vi "Test Simple Connection.vi"() -> ()   [LabVIEW 2013]
uses:
  <vilib>/LabVIEW Open Source Project/MQTT Control Packets/Control Packets/CONNECT/CONNECT.lvclass
  <vilib>/LabVIEW Open Source Project/MQTT Control Packets/Control Packets/CONNACK/Connect Return Code -- enum.ctl
  MQTT_Connection/Connection/Connection.lvclass
  <vilib>/LabVIEW Open Source Project/MQTT Control Packets/Control Packets/PUBLISH/PUBLISH.lvclass
  <vilib>/LabVIEW Open Source Project/MQTT Control Packets/Control Packets/ControlPacket/ControlPacket.lvclass
  <vilib>/LabVIEW Open Source Project/MQTT Control Packets/Control Packets/CONNACK/CONNACK.lvclass
  <vilib>/LabVIEW Open Source Project/MQTT Control Packets/Control Packets/ControlPacket/ControlPacket.lvclass/ControlPacket.ctl
  <vilib>/LabVIEW Open Source Project/MQTT Control Packets/Control Packets/DISCONNECT/DISCONNECT.lvclass
  <vilib>/LabVIEW Open Source Project/MQTT Control Packets/Control Packets/MQTT_311/MQTTVersion.lvclass
  MQTT_TCP/Connection/TCPConnection.lvclass
  MQTT_LocalQueue/Connection/LocalQueueConnection.lvclass
panel:
  in  "Channel Under Test":T1(ring)
  in  "Range (max)":dbl=1.0
  out "randomNumber":dbl
  out "Topic":string
  out "connected":bool
  in  "Connect to Server":bool
  out "client":errorcluster
  out "server":errorcluster
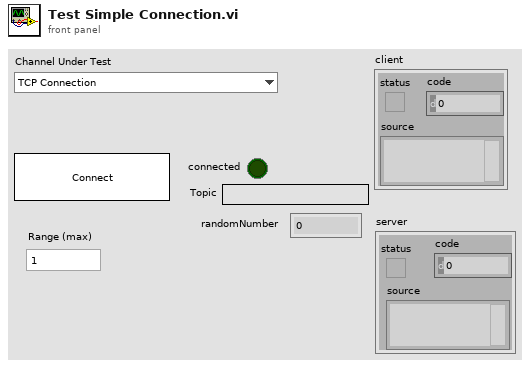
[diagram p1: front panel]
types:
  T1 = enum16{"TCP Connection", "Local Queue Connection"}
  T2 = cluster{"Packet":refnum<class "ControlPacket.lvclass">, "Direction":enum16{"In", "Out"}}
  T3 = cluster{"connected":refnum<user-event>, "Incoming Message":refnum<user-event>}
  T4 = cluster{"Connection":refnum<class "Connection.lvclass">, "Public Events":cluster{"connected":refnum<user-event>, "Incoming Message":refnum<user-event>}, "Payload":refnum<queue>}
  T5 = typedef "MQTT_Control_Packets.lvlib/CONNACK.lvclass/Connect Return Code -- enum.ctl" = enum16{"Connection accepted", "Unacceptable protocol version", "Identifier Rejected", "Server Unavailable", "Bad Username or Password", "Not Authorized"}
  T6 = enum16{"Standard", "Buffered", "CRLF", "Immediate"}
  T7 = typedef "MQTT_Control_Packets.lvlib/ControlPacket.lvclass/Control Packet Type -- enum.ctl" = enum16{"Reserved", "CONNECT", "CONNACK", "PUBLISH", "PUBACK", "PUBREC", "PUBREL", "PUBCOMP", "SUBSCRIBE", "SUBACK", "UNSUBSCRIBE", "UNSUBACK", "PINGREQ", "PINGRESP", "DISCONNECT", "AUTH"}
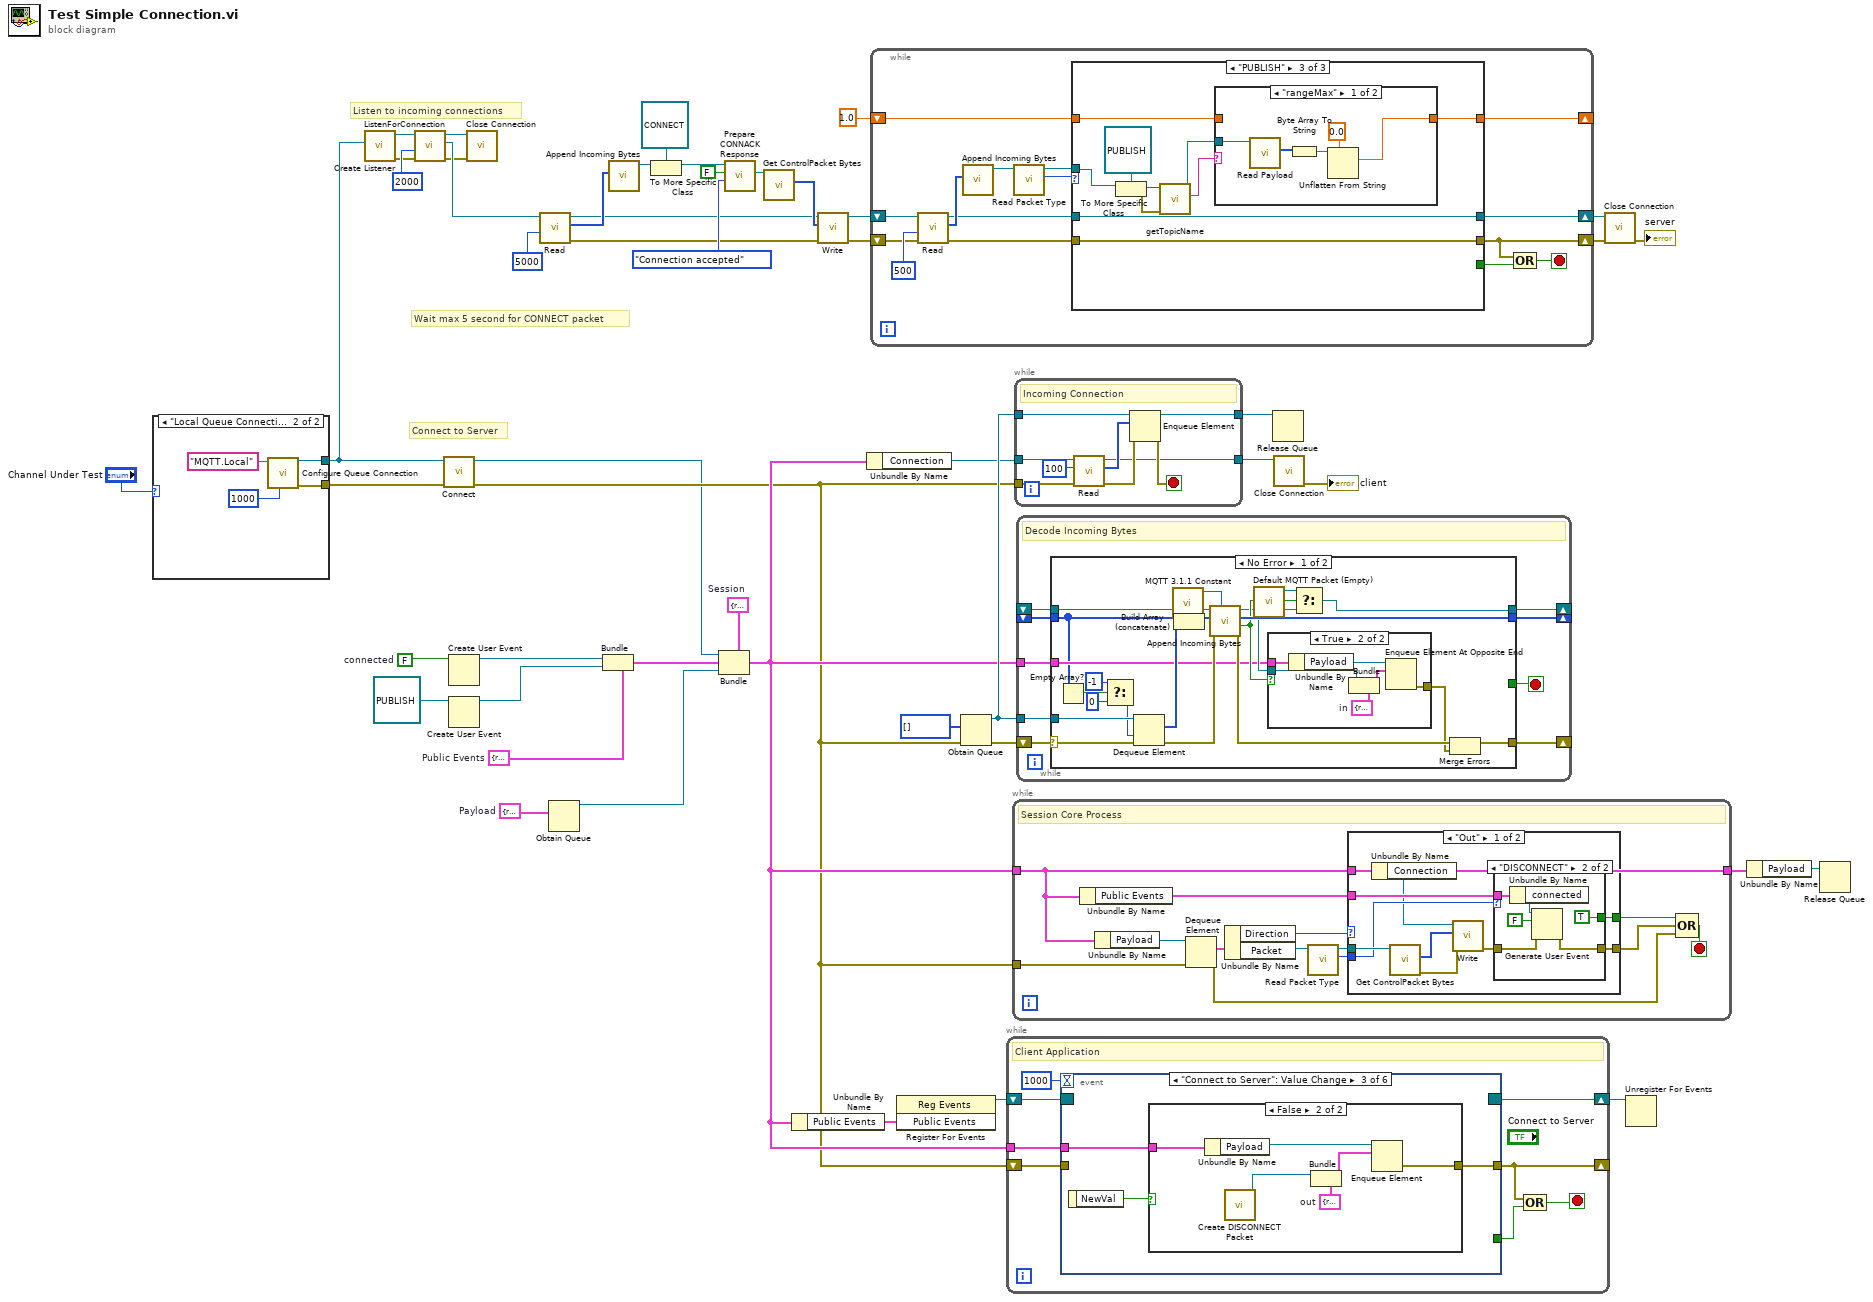
[diagram p0: block diagram]
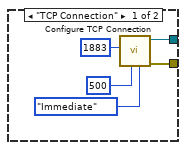
[diagram p2: hidden frame]
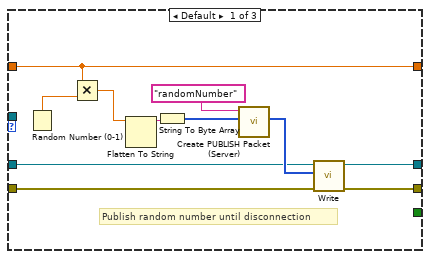
[diagram p3: hidden frame]
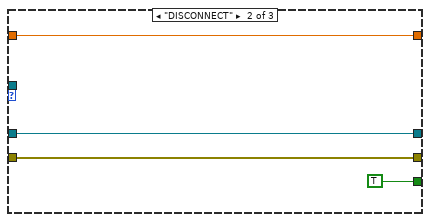
[diagram p4: hidden frame]
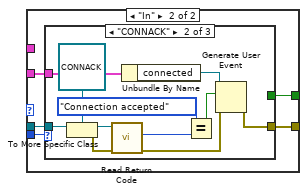
[diagram p7: hidden frame]
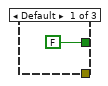
[diagram p8: hidden frame]
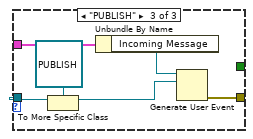
[diagram p9: hidden frame]
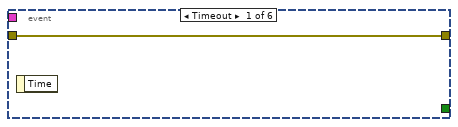
[diagram p10: hidden frame]
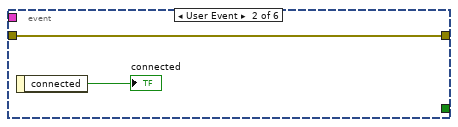
[diagram p11: hidden frame]
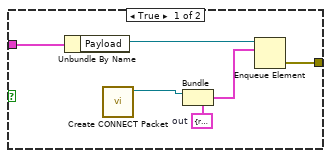
[diagram p12: hidden frame]
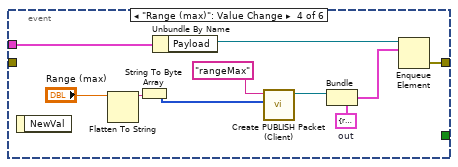
[diagram p13: hidden frame]
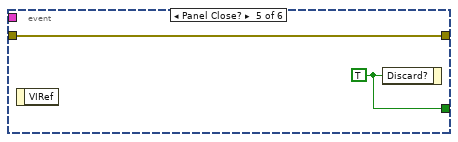
[diagram p14: hidden frame]
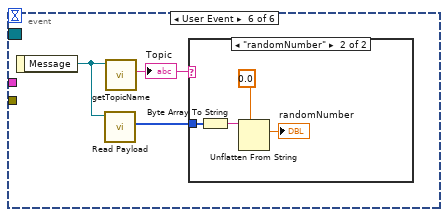
[diagram p15: hidden frame]
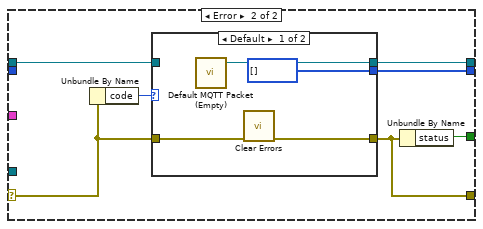
[diagram p18: hidden frame]
diagram:
  w21 = T2 {"Packet"=refnum, "Direction"=enum."In"}  # Payload
  w34 = T3 {"connected"=refnum, "Incoming Message"=refnum}  # Public Events
  w35 = FALSE  # connected
  w37 = T4 {"Connection"=refnum, "Public Events"={"connected"=refnum, "Incoming Message"=refnum}, "Payload"=refnum}  # Session
  # "Connect to Server"
  # "Listen to incoming connections"
  # "Wait max 5 second for CONNECT packet"
  n1 = case shown="\"Local Queue Connection\"" "Channel Under Test" {
    tunnel: [w52 w57] -> w9
    tunnel: [w51 w58] -> w2
    frame "TCP Connection" {
      n2 = call "Configure TCP Connection.vi"("Read Mode (Immediate)"=T6."Immediate" ("mode (standard)"), "timeout (5000ms)"=500 ("timeout (100ms)"), "remote port (80)"=u16 1883) -> ("error out"=w52:errorcluster, "TCPConnection"=w51:refnum<class "TCPConnection.lvclass">)  [unwired: 7 in]
    }
    frame "Local Queue Connection" {
      n3 = call "Configure Queue Connection.vi"("timeout (500 ms)"=1000 ("timeout (100ms)"), "Queue Name"="MQTT.Local") -> ("error out"=w57:errorcluster, "LocalQueueConnection"=w58:refnum<class "LocalQueueConnection.lvclass">)  [unwired: 8 in]
    }
  }
  n4 = call "Create Listener.vi"("Connection Configuration"=w2) -> ("error out"=w4:errorcluster, "Listener"=w8:refnum<class "Connection.lvclass">)  [unwired: 9 in]
  n5 = call "ListenForConnection.vi"("error in (no error)"=w4, "timeout (ms)"=2000 ("bytes to read (100)"), "Listener"=w8) -> ("error out"=w3:errorcluster, "Connection"=w5:refnum<class "Connection.lvclass">, "Listener out"=w6:refnum<class "Connection.lvclass">)  [unwired: 5 in, 1 out]
  n6 = call "Connect.vi"("error in (no error)"=w9, "Connection in"=w2) -> ("error out"=w11:errorcluster, "Connection out"=w10:refnum<class "Connection.lvclass">)  [unwired: 8 in]
  n7 = Create User Event(user event datatype=w35) -> (user event=w36:refnum<user-event>)  [unwired: 1 in, 1 out]
  n8 = Create User Event(user event datatype=refnum<class "PUBLISH.lvclass"> refnum ("Message")) -> (user event=w26:refnum<user-event>)  [unwired: 1 in, 1 out]
  n9 = call "Close Connection.vi"("error in (no error)"=w3, "Connection in"=w6) -> ()  [unwired: 8 in, 2 out]
  n10 = call "Read.vi"("timeout (1000 ms)"=5000 ("bytes to read (100)"), "TCPConnection in"=w5) -> ("error out"=w14:errorcluster, "Bytes"=w13:u8[], "TCPConnection out"=w12:refnum<class "Connection.lvclass">)  [unwired: 5 in, 2 out]
  n11 = Obtain Queue(element data type=w21) -> (queue out=w19:refnum<queue>)  [unwired: 4 in, 2 out]
  n12 = Bundle(cluster=w34, "connected"=w36, "Incoming Message"=w26) -> (w20:T3)
  n13 = call <vilib>:"Append Incoming Bytes.vi"("Incoming Packets"=w13) -> ("ControlPacket"=w50:refnum<class "ControlPacket.lvclass">)  [unwired: 7 in, 3 out]
  n14 = To More Specific Class(target class=refnum<class "CONNECT.lvclass"> refnum ("CONNECT in"), reference=w50) -> (specific class reference=w49:refnum<class "CONNECT.lvclass">)  [unwired: 1 in, 1 out]
  n15 = Bundle(cluster=w37, "Connection"=w10, "Public Events"=w20, "Payload"=w19) -> (w17:T4)
  n16 = call-dynamic "Prepare CONNACK Response.vi"("Return Code"=Connect_Return_Code_--_enum."Connection accepted", "Session Present"=FALSE, "CONNECT in"=w49) -> ("CONNACK response"=w46:refnum<class "CONNACK.lvclass">)  [unwired: 5 in, 3 out]
  n17 = call <vilib>:"Get ControlPacket Bytes.vi"("ControlPacket"=w46) -> ("Bytes Stream"=w47:u8[])  [unwired: 7 in, 3 out]
  n18 = Unbundle By Name(w17) -> ("Public Events"=w33:T3)
  n19 = call "Write.vi"("error in (no error)"=w14, "Bytes"=w47, "Connection in"=w12) -> ("error out"=w24:errorcluster, "Connection"=w25:refnum<class "Connection.lvclass">)  [unwired: 7 in]
  n20 = Unbundle By Name(w17) -> ("Connection"=w16:refnum<class "Connection.lvclass">)
  n21 = while {
    shift-right: [w66] -> w23
    shift-left: w25 -> [w71]
    shift-right: [w63] -> w22
    shift-left: w24 -> [w70]
    shift-right: [w61] -> _
    shift-left: 1.0 -> [w62]
    stop <- w64 stop-if-true
    n22 = call "Read.vi"("error in (no error)"=w70, "timeout (1000 ms)"=500 ("bytes to read (100)"), "TCPConnection in"=w71) -> ("error out"=w67:errorcluster, "Bytes"=w74:u8[], "TCPConnection out"=w68:refnum<class "Connection.lvclass">)  [unwired: 4 in, 2 out]
    n23 = call <vilib>:"Append Incoming Bytes.vi"("Incoming Packets"=w74) -> ("ControlPacket"=w73:refnum<class "ControlPacket.lvclass">)  [unwired: 7 in, 3 out]
    n24 = call <vilib>:"Read Packet Type.vi"("ControlPacket in"=w73) -> ("Control Packet Type"=w69:T7, "ControlPacket out"=w60:refnum<class "ControlPacket.lvclass">)  [unwired: 9 in]
    n25 = case shown="\"PUBLISH\"" w69 {
      tunnel: w68 -> [w81 w89 w99]
      tunnel: w67 -> [w78 w88 w98]
      tunnel: [w80 w89 w99] -> w66
      tunnel: [w79 w88 w98] -> w63
      tunnel: [_ TRUE _] -> w65
      tunnel: w62 -> [w75 w86 w92]
      tunnel: [w75 w86 w91] -> w61
      tunnel: w60 -> [_ _ w96]
      frame Default {
        # "Publish random number until disconnection"
        n26 = Random Number (0-1)() -> (number: 0 to 1=w77:dbl)
        n27 = Multiply(x=w75, y=w77) -> (x*y=w76:dbl)
        n28 = Flatten To String(anything=w76) -> (data string=w83:string)  [unwired: 3 in, 2 out]
        n29 = String To Byte Array(string=w83) -> (unsigned byte array=w84:u8[])
        n30 = call <vilib>:"Create PUBLISH Packet (Server).vi"("Payload"=w84, "Topic Name"="randomNumber") -> ("Bytes Stream"=w85:u8[])  [unwired: 6 in, 3 out]
        n31 = call "Write.vi"("error in (no error)"=w78, "Bytes"=w85, "Connection in"=w81) -> ("error out"=w79:errorcluster, "Connection"=w80:refnum<class "Connection.lvclass">)  [unwired: 7 in]
      }
      frame "DISCONNECT" {
      }
      frame "PUBLISH" {
        n32 = To More Specific Class(target class=refnum<class "PUBLISH.lvclass"> refnum ("event data"), reference=w96) -> (specific class reference=w94:refnum<class "PUBLISH.lvclass">, error out=w95:errorcluster)  [unwired: 1 in]
        n33 = call <vilib>:"getTopicName.vi"("error in (no error)"=w95, "PUBLISH in"=w94) -> ("Topic"=w93:string, "PUBLISH out"=w90:refnum<class "PUBLISH.lvclass">)  [unwired: 7 in, 1 out]
        n34 = case shown="\"rangeMax\"" w93 {
          tunnel: w92 -> [_ w105]
          tunnel: [w100 w105] -> w91
          tunnel: w90 -> [w104 _]
          frame "rangeMax" {
            n35 = call <vilib>:"Read Payload.vi"("ControlPacket in"=w104) -> ("Payload"=w101:u8[])  [unwired: 9 in, 1 out]
            n36 = Byte Array To String(unsigned byte array=w101) -> (string=w102:string)
            n37 = Unflatten From String(type=0.0, binary string=w102) -> (value=w100:dbl)  [unwired: 3 in, 2 out]
          }
          frame Default {
          }
        }
      }
    }
    n38 = Compound Arithmetic op=OR(w63, w65) -> (w64:bool)
  }
  n39 = register-events(w33) -> (reference out=w39:refnum<event-registration>)  [unwired: 2 in, 1 out]
  n40 = Obtain Queue(element data type=u8[] [] ("Remaining Packets"), error in (no error)=w11) -> (queue out=w43:refnum<queue>, error out=w41:errorcluster)  [unwired: 3 in, 1 out]
  n41 = while {
    shift-right: [w111] -> w38
    shift-left: w39 -> [w112]
    shift-right: [w109] -> _
    shift-left: w11 -> [w110]
    tunnel: w17 -> [w107]
    stop <- w108 stop-if-true
    # "Client Application"
    n42 = event shown="[2] \"Connect to Server\": Value Change" {
      selector: w112 -> [_ _ _ _ _ _]
      dyn-events: [_ _ _ _ _ _] -> w111
      timeout: 1000 -> [_ _ _ _ _ _]
      tunnel: [_ _ _ _ w143 _] -> w106
      tunnel: [w114 w116 w117 w140 w142 _] -> w109
      tunnel: w110 -> [w114 w116 _ _ w142 _]
      tunnel: w107 -> [_ _ w118 w141 _ _]
      event Timeout {
        n43 = event-data() -> ()  [unwired: 1 in, 1 out]
      }
      event User Event {
        n44 = event-data() -> ("connected"=→"connected":bool)  [unwired: 1 in]
      }
      event "Connect to Server": Value Change {
        n45 = event-data() -> ("NewVal"=w119:bool)  [unwired: 1 in]
        n46 = case shown="False" w119 {
          tunnel: w118 -> [w125 w131]
          tunnel: [w123 w129] -> w117
          frame True {
            w122 = T2 {"Packet"=refnum, "Direction"=enum."Out"}  # out
            n47 = Unbundle By Name(w125) -> ("Payload"=w124:refnum<queue>)
            n48 = call <vilib>:"Create CONNECT Packet.vi"() -> ("CONNECT"=w121:refnum<class "CONNECT.lvclass">)  [unwired: 9 in, 2 out]
            n49 = Bundle(cluster=w122, "Packet"=w121) -> (w120:T2)  [unwired: 1 in]
            n50 = Enqueue Element(queue=w124, element=w120) -> (error out=w123:errorcluster)  [unwired: 2 in, 2 out]
          }
          frame False {
            w126 = T2 {"Packet"=refnum, "Direction"=enum."Out"}  # out
            n51 = Unbundle By Name(w131) -> ("Payload"=w130:refnum<queue>)
            n52 = call <vilib>:"Create DISCONNECT Packet.vi"() -> ("DISCONNECT"=w128:refnum<class "DISCONNECT.lvclass">)  [unwired: 9 in, 2 out]
            n53 = Bundle(cluster=w126, "Packet"=w128) -> (w127:T2)  [unwired: 1 in]
            n54 = Enqueue Element(queue=w130, element=w127) -> (error out=w129:errorcluster)  [unwired: 2 in, 2 out]
          }
        }
      }
      event "Range (max)": Value Change {
        w138 = T2 {"Packet"=refnum, "Direction"=enum."Out"}  # out
        n55 = event-data() -> ()  [unwired: 1 in, 1 out]
        n56 = Flatten To String(anything="Range (max)") -> (data string=w134:string)  [unwired: 3 in, 2 out]
        n57 = String To Byte Array(string=w134) -> (unsigned byte array=w133:u8[])
        n58 = Unbundle By Name(w141) -> ("Payload"=w139:refnum<queue>)
        n59 = call <vilib>:"Create PUBLISH Packet (Client).vi"("Payload"=w133, "Topic Name"="rangeMax") -> ("PUBLISH"=w136:refnum<class "PUBLISH.lvclass">)  [unwired: 6 in, 3 out]
        n60 = Bundle(cluster=w138, "Packet"=w136) -> (w137:T2)  [unwired: 1 in]
        n61 = Enqueue Element(queue=w139, element=w137) -> (error out=w140:errorcluster)  [unwired: 2 in, 2 out]
      }
      event Panel Close? {
        w143 = TRUE ("Discard?")
        n62 = event-data() -> ()  [unwired: 1 in, 1 out]
        n63 = event-data("Discard?"=w143) -> ()  [unwired: 1 in, 1 out]
      }
      event User Event {
        n64 = event-data() -> ("Message"=w146:refnum<class "PUBLISH.lvclass">)  [unwired: 1 in]
        n65 = call <vilib>:"Read Payload.vi"("ControlPacket in"=w146) -> ("Payload"=w144:u8[])  [unwired: 9 in, 1 out]
        n66 = call <vilib>:"getTopicName.vi"("PUBLISH in"=w146) -> ("Topic"=w145:string)  [unwired: 8 in, 2 out]
        "Topic" <- w145
        n67 = case shown="\"randomNumber\"" w145 {
          tunnel: w144 -> [_ w149]
          frame "False", Default {
          }
          frame "randomNumber" {
            n68 = Byte Array To String(unsigned byte array=w149) -> (string=w148:string)
            n69 = Unflatten From String(type=0.0, binary string=w148) -> (value=→"randomNumber":dbl)  [unwired: 3 in, 2 out]
          }
        }
      }
    }
    n70 = Compound Arithmetic op=OR(w109, w106) -> (w108:bool)
  }
  n71 = while {
    tunnel: w17 -> [w152]
    tunnel: [w152] -> w32
    tunnel: w11 -> [w161]
    stop <- w157 stop-if-true
    # "Session Core Process"
    n72 = Unbundle By Name(w152) -> ("Public Events"=w151:T3)
    n73 = Unbundle By Name(w152) -> ("Payload"=w156:refnum<queue>)
    n74 = Dequeue Element(queue=w156, error in (no error)=w161) -> (element=w155:T2, error out=w158:errorcluster)  [unwired: 1 in, 2 out]
    n75 = Unbundle By Name(w155) -> ("Direction"=w153:enum16{"In", "Out"}, "Packet"=w154:refnum<class "ControlPacket.lvclass">)
    n76 = call <vilib>:"Read Packet Type.vi"("ControlPacket in"=w154) -> ("Control Packet Type"=w163:T7, "ControlPacket out"=w162:refnum<class "ControlPacket.lvclass">)  [unwired: 9 in]
    n77 = case shown="\"Out\"" w153 {
      tunnel: w163 -> [w169 w185]
      tunnel: w162 -> [w171 w184]
      tunnel: [w173 w183] -> w160
      tunnel: [w172 w182] -> w159
      tunnel: w152 -> [w170 _]
      tunnel: w151 -> [w168 w181]
      frame "Out" {
        n78 = Unbundle By Name(w170) -> ("Connection"=w167:refnum<class "Connection.lvclass">)
        n79 = call <vilib>:"Get ControlPacket Bytes.vi"("ControlPacket"=w171) -> ("error out"=w165:errorcluster, "Bytes Stream"=w166:u8[])  [unwired: 7 in, 2 out]
        n80 = call "Write.vi"("error in (no error)"=w165, "Bytes"=w166, "Connection in"=w167) -> ("error out"=w164:errorcluster)  [unwired: 7 in, 1 out]
        n81 = case shown="\"DISCONNECT\"" w169 {
          tunnel: [_ TRUE] -> w173
          tunnel: [w174 w178] -> w172
          tunnel: w164 -> [w174 w177]
          tunnel: w168 -> [_ w176]
          frame Default {
          }
          frame "DISCONNECT" {
            n82 = Unbundle By Name(w176) -> ("connected"=w175:refnum<user-event>)
            n83 = Generate User Event(user event=w175, event data cluster=FALSE ("event data"), error in=w177) -> (error out=w178:errorcluster)  [unwired: 1 in, 1 out]
          }
        }
      }
      frame "In" {
        n84 = case shown="\"CONNACK\"" w185 {
          tunnel: w184 -> [_ w197 w202]
          tunnel: [_ w192 w203] -> w182
          tunnel: [FALSE _ _] -> w183
          tunnel: w181 -> [_ w187 w199]
          frame Default {
          }
          frame "CONNACK" {
            n85 = To More Specific Class(target class=refnum<class "CONNACK.lvclass"> refnum ("CONNACK in"), reference=w197) -> (specific class reference=w195:refnum<class "CONNACK.lvclass">, error out=w190:errorcluster)  [unwired: 1 in]
            n86 = call <vilib>:"Read Return Code.vi"("error in (no error)"=w190, "CONNACK in"=w195) -> ("error out"=w191:errorcluster, "Return Code"=w194:T5)  [unwired: 7 in, 1 out]
            n87 = Unbundle By Name(w187) -> ("connected"=w188:refnum<user-event>)
            n88 = Equal?(x=Connect_Return_Code_--_enum."Connection accepted", y=w194) -> (x = y?=w193:bool)
            n89 = Generate User Event(user event=w188, event data cluster=w193, error in=w191) -> (error out=w192:errorcluster)  [unwired: 1 in, 1 out]
          }
          frame "PUBLISH" {
            n90 = To More Specific Class(target class=refnum<class "PUBLISH.lvclass"> refnum ("event data"), reference=w202) -> (specific class reference=w200:refnum<class "PUBLISH.lvclass">)  [unwired: 1 in, 1 out]
            n91 = Unbundle By Name(w199) -> ("Incoming Message"=w198:refnum<user-event>)
            n92 = Generate User Event(user event=w198, event data cluster=w200) -> (error out=w203:errorcluster)  [unwired: 2 in, 1 out]
          }
        }
      }
    }
    n93 = Compound Arithmetic op=OR(w160, w159, w158) -> (w157:bool)
  }
  n94 = while {
    tunnel: w43 -> [w212]
    tunnel: w16 -> [w209]
    tunnel: [w204] -> w40
    tunnel: [w211] -> w30
    tunnel: w11 -> [w207]
    stop <- w210 stop-if-true
    # "Incoming Connection"
    n95 = call "Read.vi"("error in (no error)"=w207, "bytes to read (100)"=100, "TCPConnection in"=w209) -> ("error out"=w206:errorcluster, "Bytes"=w205:u8[], "TCPConnection out"=w204:refnum<class "Connection.lvclass">)  [unwired: 4 in, 2 out]
    n96 = Enqueue Element(queue=w212, element=w205, error in (no error)=w206) -> (queue out=w211:refnum<queue>, error out=w210:errorcluster)  [unwired: 1 in, 1 out]
  }
  n97 = while {
    shift-right: [w219] -> _
    shift-left: _ -> [w218]
    shift-right: [w217] -> _
    shift-left: w41 -> [w216]
    shift-right: [w220] -> _
    shift-left: _ -> [w221]
    tunnel: w17 -> [w213]
    tunnel: w43 -> [w214]
    stop <- w215 stop-if-true
    # "Decode Incoming Bytes"
    n98 = case shown="No Error" w216 {
      selector: w216 -> [w236 w253]
      tunnel: w221 -> [w242 w251]
      tunnel: [w232 w255] -> w220
      tunnel: [w240 w254] -> w219
      tunnel: w218 -> [w223 _]
      tunnel: [w233 w250] -> w217
      tunnel: [_ w249] -> w215
      tunnel: w214 -> [w239 _]
      tunnel: w213 -> [w227 _]
      frame No Error {
        # "No Error"
        n99 = Empty Array?(array=w223) -> (empty?=w226:bool)
        n100 = Select(t=-1 ("timeout in ms (-1)"), s=w226, f=0) -> (s? t:f=w222:i32)
        n101 = Dequeue Element(queue=w239, timeout in ms (-1)=w222, error in (no error)=w236) -> (element=w238:u8[], error out=w235:errorcluster)  [unwired: 2 out]
        n102 = call <vilib>:"MQTT 3.1.1 Constant.vi"() -> ("MQTT 3.1.1"=w241:refnum<class "MQTTVersion.lvclass">)  [unwired: 11 in]
        n103 = Build Array (concatenate)(w223, w238) -> (w237:u8[])
        n104 = call <vilib>:"Append Incoming Bytes.vi"("MQTT Version (3.1.1)"=w241, "error in (no error)"=w235, "Incoming Packets"=w237, "Incomplete ControlPacket"=w242) -> ("error out"=w234:errorcluster, "Complete Packet"=w230:bool, "Remaining Packets"=w240:u8[], "ControlPacket"=w229:refnum<class "ControlPacket.lvclass">)  [unwired: 4 in]
        n105 = call <vilib>:"Default MQTT Packet (Empty).vi"() -> ("No Packet"=w231:refnum<class "ControlPacket.lvclass">)  [unwired: 11 in]
        n106 = case shown="True" w230 {
          tunnel: [_ w248] -> w228
          tunnel: w229 -> [_ w245]
          tunnel: w227 -> [_ w243]
          frame False {
            # "No Packet received"
          }
          frame True {
            w247 = T2 {"Packet"=refnum, "Direction"=enum."In"}  # in
            # "Packet Received"
            n107 = Unbundle By Name(w243) -> ("Payload"=w244:refnum<queue>)
            n108 = Bundle(cluster=w247, "Packet"=w245) -> (w246:T2)  [unwired: 1 in]
            n109 = Enqueue Element At Opposite End(queue=w244, element=w246) -> (error out=w248:errorcluster)  [unwired: 2 in, 2 out]
          }
        }
        n110 = Select(t=w231, s=w230, f=w229) -> (s? t:f=w232:refnum<class "ControlPacket.lvclass">)
        n111 = Merge Errors(w234, w228) -> (w233:errorcluster)
      }
      frame Error {
        # "Handle Error"
        n112 = Unbundle By Name(w253) -> ("code"=w252:i32)
        n113 = case shown="Default" w252 {
          tunnel: [w256 w261] -> w255
          tunnel: w253 -> [w259 w260]
          tunnel: [w258 w260] -> w250
          tunnel: [u8[] [] ("Remaining Packets") _] -> w254
          tunnel: w251 -> [_ w261]
          frame Default {
            # "Malformed Packet"
            n114 = call <vilib>:"Default MQTT Packet (Empty).vi"() -> ("No Packet"=w256:refnum<class "ControlPacket.lvclass">)  [unwired: 11 in]
            n115 = call <vilib>:"Clear Errors.vi"("error in (no error)"=w259) -> ("error out"=w258:errorcluster)  [unwired: 6 in]
          }
          frame 1, 66, 1556 {
          }
        }
        n116 = Unbundle By Name(w250) -> ("status"=w249:bool)
      }
    }
  }
  n117 = Release Queue(queue=w30) -> ()  [unwired: 2 in, 3 out]
  n118 = call "Close Connection.vi"("Connection in"=w40) -> ("error out"=→"client":errorcluster)  [unwired: 9 in, 1 out]
  n119 = call "Close Connection.vi"("error in (no error)"=w22, "Connection in"=w23) -> ("error out"=→"server":errorcluster)  [unwired: 8 in, 1 out]
  n120 = Unregister For Events(event registration refnum=w38) -> ()  [unwired: 1 in, 1 out]
  n121 = Unbundle By Name(w32) -> ("Payload"=w31:refnum<queue>)
  n122 = Release Queue(queue=w31) -> ()  [unwired: 2 in, 3 out]
